vi "Save end points.vi"(5 "section":string="Encoders", 8 "error in (no error)":errorcluster, 9 "Cluster":T1={"Encoder 1 channel A"="Encoder 1 channel A", "Encoder 1 A"=1234.0, "Encoder 1 channel B"="Encoder 1 channel B", "Encoder 1 B"=5678.0, "Encoder 2 channel A"="Encoder 2 channel A", "Encoder 2 A"=4321.0, "Encoder 2 channel B"="Encoder 2 channel B", "Encoder 2 B"=8765.0, "Encoder 3 channel A"="Encoder 3 channel A", "Encoder 3 A "=1111.0, "Encoder 3 channel B"="Encoder 3 channel B", "Encoder 3 B"=2222.0, "Encoder 4 channel A "="Encoder 3 channel B", "Encoder 4 channel B"="Encoder 3 channel B", "Encoder 4 A"=2222.0, "Encoder 4 B "=2222.0}, 10 "write file if changed (T)":bool=TRUE, 11 "start path":path=path "C:/Users/Team1699/Documents/Test.ini") -> (0 "error out":errorcluster)   [LabVIEW 2012]
uses:
  <vilib>/Utility/config.llb/Write Key (Double).vi
  <vilib>/Utility/config.llb/NI_LVConfig.lvlib
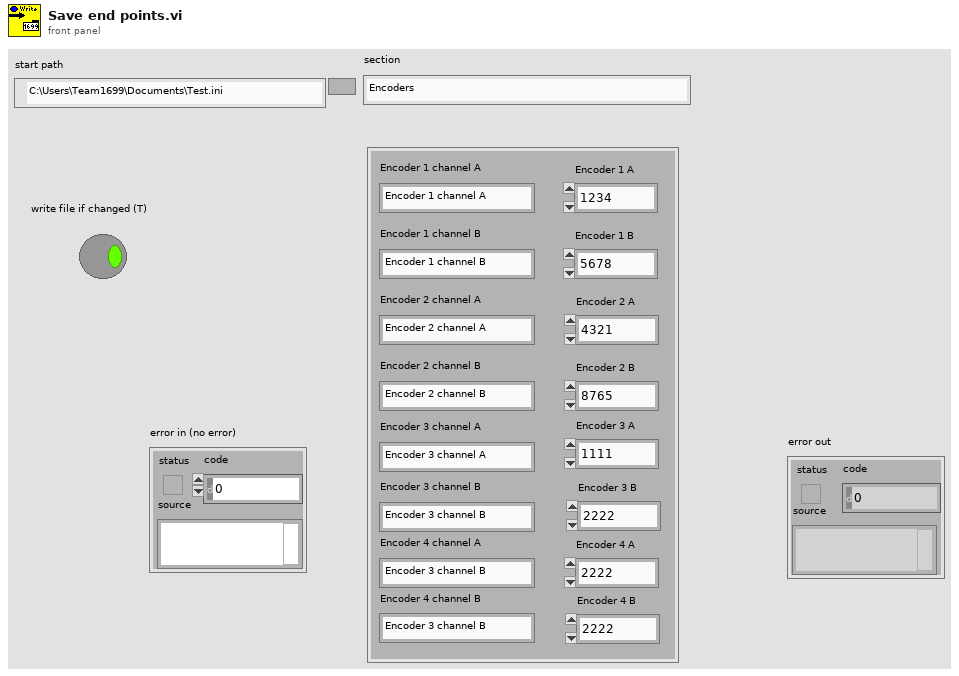
[diagram p1: front panel]
types:
  T1 = cluster{"Encoder 1 channel A":string, "Encoder 1 A":dbl, "Encoder 1 channel B":string, "Encoder 1 B":dbl, "Encoder 2 channel A":string, "Encoder 2 A":dbl, "Encoder 2 channel B":string, "Encoder 2 B":dbl, "Encoder 3 channel A":string, "Encoder 3 A ":dbl, "Encoder 3 channel B":string, "Encoder 3 B":dbl, "Encoder 4 channel A ":string, "Encoder 4 channel B":string, "Encoder 4 A":dbl, "Encoder 4 B ":dbl}
  T2 = typedef "NI_LVConfig.lvlib/Config Data RefNum.ctl" = refnum<k1>
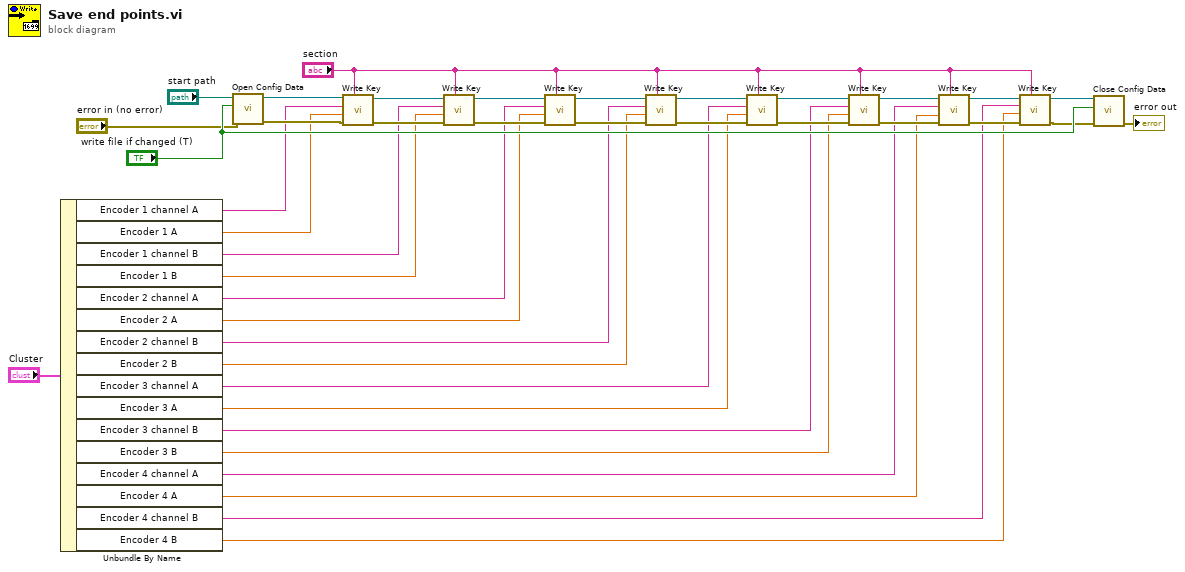
[diagram p0: block diagram]
diagram:
  n1 = Unbundle By Name("Cluster") -> ("Encoder 1 channel A"=w23:string, "Encoder 1 A"=w22:dbl, "Encoder 1 channel B"=w21:string, "Encoder 1 B"=w20:dbl, "Encoder 2 channel A"=w19:string, "Encoder 2 A"=w18:dbl, "Encoder 2 channel B"=w17:string, "Encoder 2 B"=w16:dbl, "Encoder 3 channel A"=w15:string, "Encoder 3 A"=w14:dbl, "Encoder 3 channel B"=w13:string, "Encoder 3 B"=w12:dbl, "Encoder 4 channel A"=w4:string, "Encoder 4 A"=w3:dbl, "Encoder 4 channel B"=w2:string, "Encoder 4 B"=w1:dbl)
  n2 = call <vilib>:"Open Config Data.vi"("error in (no error)"="error in (no error)", "create file if necessary (T)"="write file if changed (T)", "configuration file path"="start path") -> ("error out"=w39:errorcluster, "refnum"=w40:T2)  [unwired: 6 in, 1 out]
  n3 = call-poly <vilib>:"Write Key.vi"("section"="section", "error in (no error)"=w39, "value"=w22, "key"=w23, "refnum"=w40) -> ("error out"=w33:errorcluster, "refnum out"=w38:T2)  [unwired: 4 in, 1 out]
  n4 = call-poly <vilib>:"Write Key.vi"("section"="section", "error in (no error)"=w33, "value"=w20, "key"=w21, "refnum"=w38) -> ("error out"=w32:errorcluster, "refnum out"=w37:T2)  [unwired: 4 in, 1 out]
  n5 = call-poly <vilib>:"Write Key.vi"("section"="section", "error in (no error)"=w32, "value"=w18, "key"=w19, "refnum"=w37) -> ("error out"=w31:errorcluster, "refnum out"=w36:T2)  [unwired: 4 in, 1 out]
  n6 = call-poly <vilib>:"Write Key.vi"("section"="section", "error in (no error)"=w31, "value"=w16, "key"=w17, "refnum"=w36) -> ("error out"=w30:errorcluster, "refnum out"=w35:T2)  [unwired: 4 in, 1 out]
  n7 = call-poly <vilib>:"Write Key.vi"("section"="section", "error in (no error)"=w30, "value"=w14, "key"=w15, "refnum"=w35) -> ("error out"=w29:errorcluster, "refnum out"=w34:T2)  [unwired: 4 in, 1 out]
  n8 = call-poly <vilib>:"Write Key.vi"("section"="section", "error in (no error)"=w29, "value"=w12, "key"=w13, "refnum"=w34) -> ("error out"=w8:errorcluster, "refnum out"=w5:T2)  [unwired: 4 in, 1 out]
  n9 = call-poly <vilib>:"Write Key.vi"("section"="section", "error in (no error)"=w8, "value"=w3, "key"=w4, "refnum"=w5) -> ("error out"=w11:errorcluster, "refnum out"=w10:T2)  [unwired: 4 in, 1 out]
  n10 = call-poly <vilib>:"Write Key.vi"("section"="section", "error in (no error)"=w11, "value"=w1, "key"=w2, "refnum"=w10) -> ("error out"=w6:errorcluster, "refnum out"=w7:T2)  [unwired: 4 in, 1 out]
  n11 = call <vilib>:"Close Config Data.vi"("error in (no error)"=w6, "write file if changed (T)"="write file if changed (T)", "refnum"=w7) -> ("error out"=→"error out":errorcluster)  [unwired: 7 in, 1 out]
